vi "子VI-查看某框-不显示界面.vi"(0 "框号":dbl format="%#_13g", 1 "框组":T4(array[cluster]), 2 "临界Z值":i32, 3 "反射图原始路径":path, 4 "临界面积百分比值":dbl, 5 "预先配置的灰度阈值":dbl, 6 "穿透图原始路径":path, 7 "部位信息":string[](array[string])=["", "34.500000", "32.500000", "1121", "34", "54.955926", "分层类", "不合格", ""], 12 "产品规格":cluster{"产品长度（周长）（mm）":dbl, "产品宽度（母线长）（mm）":dbl}) -> (14 "全部检测结果":string[][](table))   [LabVIEW 2018]
uses:
  <vilib>/vision/NI_Vision_Development_Module.lvlib
panel:
  out "弥散类检测结果":string[][](table)
  out "?":string[][](table)
  in  "格式字符串 4":string="%f"
  in  "分隔符（'\\'代码显示） 3":string="\t"
  out "Particle Reports (Pixels)":T1(array[cluster]) {"Orientation" format="%.2f"; "Dimensions"."Height" format="%.2f"; "Dimensions"."Width" format="%.2f"; "Center of Mass"."Y" format="%.2f"; "Center of Mass"."X" format="%.2f"; "Bounding Rect"."Bottom" format="%.2f"; "Bounding Rect"."Right" format="%.2f"; "Bounding Rect"."Top" format="%.2f"; "Bounding Rect"."Left" format="%.2f"; "Number of Holes" format="%.2f"; "Area" format="%.2f"}
  in  "格式字符串 3":string="%f"
  in  "分隔符（'\\'代码显示） 2":string="\t"
  out "弥散缺陷个数":i32
  out "分层缺陷个数":i32
  out "合格？ 弥散类":string="fencengThreshold"
  out "合格？分层类":string="fencengThreshold"
  in  "Tab Control":T2
  out "穿透ROI":T3(plugin-control)
  out "Threshold Image":T3(plugin-control)
  out "?":T3(plugin-control)
  out "?":T3(plugin-control)
  out "Threshold Image":T3(plugin-control)
  out "Threshold Image":T3(plugin-control)
  out "面积 (pixels)":i32
  in  "格式字符串 2":string="%f"
  in  "分隔符（'\\'代码显示）":string="\t"
  # "所选区域信息"
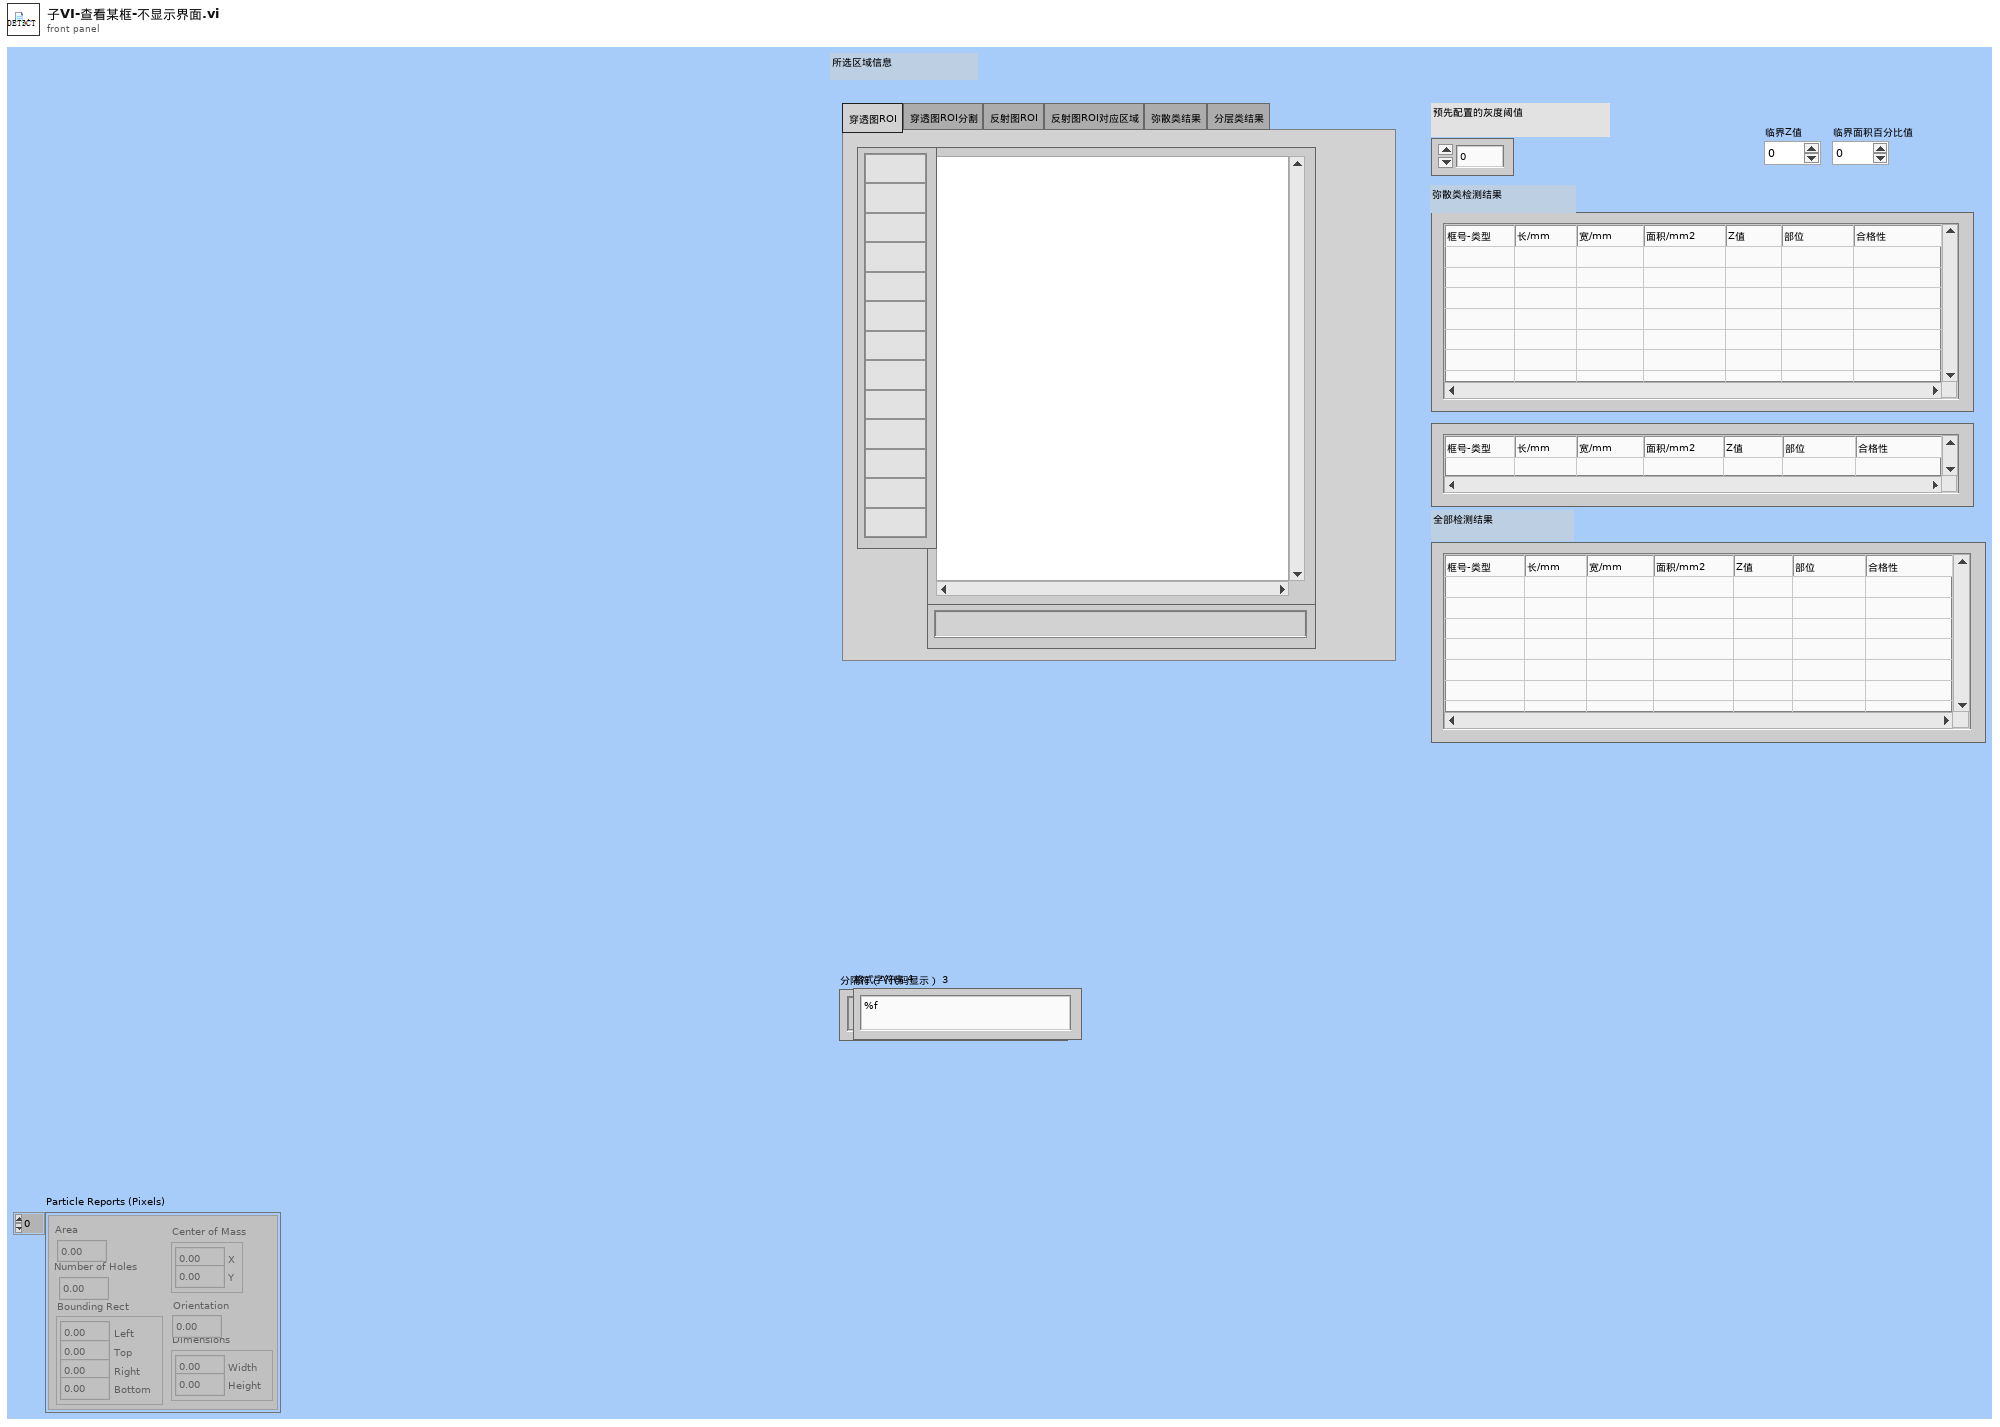
[diagram p1: front panel]
types:
  T1 = cluster{"Area":dbl, "Number of Holes":dbl, "Bounding Rect":cluster{"Left":dbl, "Top":dbl, "Right":dbl, "Bottom":dbl}, "Center of Mass":cluster{"X":dbl, "Y":dbl}, "Orientation":dbl, "Dimensions":cluster{"Width":dbl, "Height":dbl}}[]
  T2 = typedef "控件 1.ctl" = enum32{"穿透图ROI", "穿透图ROI分割", "反射图ROI", "反射图ROI对应区域", "弥散类结果", "分层类结果"}
  T3 = typedef "IMAQ Image.ctl" = refnum<image>
  T4 = cluster{"Global Rectangle":i32[], "Contours":cluster{"Contour Type":u32, "ROI Type":u32, "Points":i32[]}[]}[]
  T5 = typedef "Image Type" = u32
  T6 = cluster{"Global Rectangle":i32[], "Contours":cluster{"Contour Type":u32, "ROI Type":u32, "Points":i32[]}[]}
  T7 = cluster{"histogram":u32[], "Minimal Value":sgl, "Maximal Value":sgl, "Starting Value":sgl, "Interval Width":sgl, "Mean Value":sgl, "Standard  Variation":sgl, "Area (pixels)":i32}
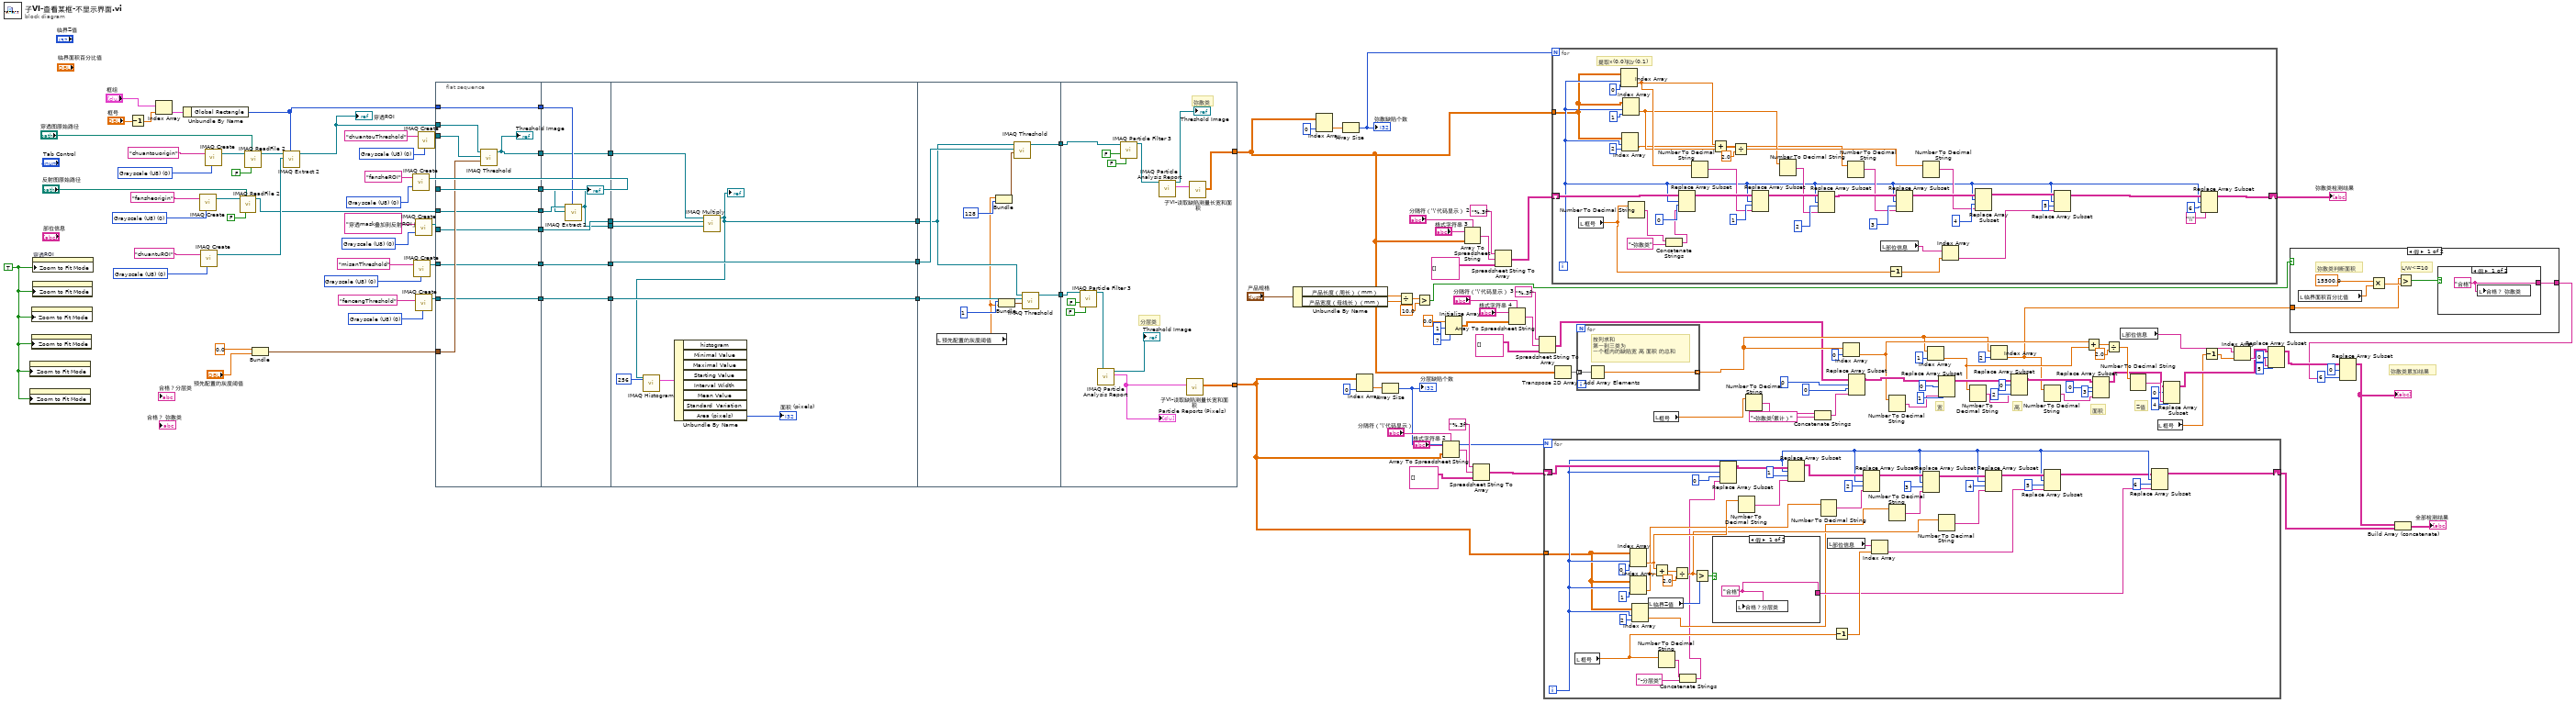
[diagram p0: block diagram]
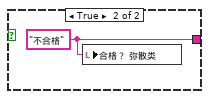
[diagram p2: hidden frame]
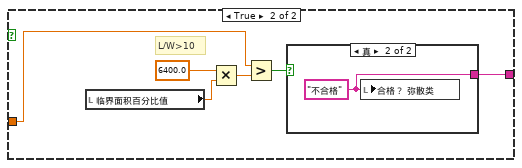
[diagram p3: hidden frame]
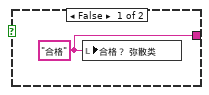
[diagram p4: hidden frame]
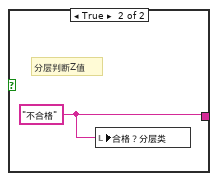
[diagram p5: hidden frame]
diagram:
  w108 = T5 0 items=["Grayscale (U8)", "Grayscale (I16)", "Grayscale (SGL)", "Complex (CSG)", "RGB (U32)", "HSL (U32)", "RGB (U64)", "Grayscale (U16)"] ("Image Type")
  w109 = T5 0 items=["Grayscale (U8)", "Grayscale (I16)", "Grayscale (SGL)", "Complex (CSG)", "RGB (U32)", "HSL (U32)", "RGB (U64)", "Grayscale (U16)"] ("Image Type")
  w110 = T5 0 items=["Grayscale (U8)", "Grayscale (I16)", "Grayscale (SGL)", "Complex (CSG)", "RGB (U32)", "HSL (U32)", "RGB (U64)", "Grayscale (U16)"] ("Image Type")
  w114 = T5 0 items=["Grayscale (U8)", "Grayscale (I16)", "Grayscale (SGL)", "Complex (CSG)", "RGB (U32)", "HSL (U32)", "RGB (U64)", "Grayscale (U16)"] ("Image Type")
  w118 = T5 0 items=["Grayscale (U8)", "Grayscale (I16)", "Grayscale (SGL)", "Complex (CSG)", "RGB (U32)", "HSL (U32)", "RGB (U64)", "Grayscale (U16)"] ("Image Type")
  w129 = T5 0 items=["Grayscale (U8)", "Grayscale (I16)", "Grayscale (SGL)", "Complex (CSG)", "RGB (U32)", "HSL (U32)", "RGB (U64)", "Grayscale (U16)"] ("Image Type")
  w102 = T5 0 items=["Grayscale (U8)", "Grayscale (I16)", "Grayscale (SGL)", "Complex (CSG)", "RGB (U32)", "HSL (U32)", "RGB (U64)", "Grayscale (U16)"] ("Image Type")
  w133 = T5 0 items=["Grayscale (U8)", "Grayscale (I16)", "Grayscale (SGL)", "Complex (CSG)", "RGB (U32)", "HSL (U32)", "RGB (U64)", "Grayscale (U16)"] ("Image Type")
  w141 = TRUE ("Zoom to Fit Mode")
  # "弥散类累加结果"
  # "Z值"
  # "面积"
  # "高"
  # "宽"
  n1 = property class="ImageControl"("Zoom to Fit Mode"=w141) -> ()  [unwired: 2 in, 2 out]
  n2 = property class="ImageControl"("Zoom to Fit Mode"=w141) -> ()  [unwired: 2 in, 2 out]
  n3 = property class="ImageControl"("Zoom to Fit Mode"=w141) -> ()  [unwired: 2 in, 2 out]
  n4 = property class="ImageControl"("Zoom to Fit Mode"=w141) -> ()  [unwired: 2 in, 2 out]
  n5 = property class="ImageControl"("Zoom to Fit Mode"=w141) -> ()  [unwired: 2 in, 2 out]
  n6 = property on="穿透ROI" class="ImageControl"("Zoom to Fit Mode"=w141) -> ()  [unwired: 2 in, 2 out]
  n7 = Decrement(x="框号") -> (x-1=w135:dbl)
  n8 = Index Array(array="框组", index=w135) -> (element=w136:T6)
  n9 = Unbundle By Name(w136) -> ("Global Rectangle"=w101:i32[])
  n10 = call "IMAQ Create"("Image Name"="fansheorigin", "Image Type"=w114) -> ("New Image"=w113:T3)  [unwired: 3 in, 1 out]
  n11 = call "IMAQ Create"("Image Name"="chuantuROI", "Image Type"=w118) -> ("New Image"=w117:T3)  [unwired: 3 in, 1 out]
  n12 = call "IMAQ Create"("Image Name"="chuantouorigin", "Image Type"=w133) -> ("New Image"=w120:T3)  [unwired: 3 in, 1 out]
  n13 = call "IMAQ ReadFile 2"("Use File Path Image Type"=FALSE, "File Path"="反射图原始路径", "Image"=w113) -> ("Image Out"=w97:T3)  [unwired: 4 in, 4 out]
  n14 = call "IMAQ ReadFile 2"("Use File Path Image Type"=FALSE, "File Path"="穿透图原始路径", "Image"=w120) -> ("Image Out"=w121:T3)  [unwired: 4 in, 4 out]
  n15 = Bundle(0.0, "预先配置的灰度阈值"="预先配置的灰度阈值") -> (w76:cluster{dbl, "预先配置的灰度阈值":dbl})  [unwired: 1 in]
  n16 = call "IMAQ Extract 2"("Optional Rectangle"=w101, "Image Dst"=w117, "Image Src"=w121) -> ("Image Dst Out"=w99:T3)  [unwired: 7 in, 1 out]
  "穿透ROI" <- w99
  n17 = call "IMAQ Create"("Image Name"="fansheROI", "Image Type"=w102) -> ("New Image"=w98:T3)  [unwired: 3 in, 1 out]
  n18 = call "IMAQ Create"("Image Name"="misanThreshold", "Image Type"=w108) -> ("New Image"=w84:T3)  [unwired: 3 in, 1 out]
  n19 = call "IMAQ Create"("Image Name"="穿透mask叠加到反射ROI上", "Image Type"=w129) -> ("New Image"=w92:T3)  [unwired: 3 in, 1 out]
  n20 = call "IMAQ Create"("Image Name"="fencengThreshold", "Image Type"=w109) -> ("New Image"=w82:T3)  [unwired: 3 in, 1 out]
  n21 = call "IMAQ Create"("Image Name"="chuantouThreshold", "Image Type"=w110) -> ("New Image"=w100:T3)  [unwired: 3 in, 1 out]
  n22 = flat-sequence {
    tunnel: w101 -> [w151]
    tunnel: w100 -> [w150]
    tunnel: w99 -> [w149]
    tunnel: w76 -> [w148]
    tunnel: w98 -> [w147]
    tunnel: w97 -> [w146]
    tunnel: [w151] -> w96
    tunnel: [w147] -> w95
    tunnel: [w146] -> w94
    tunnel: [w145] -> w93
    tunnel: w92 -> [w145]
    tunnel: [w144] -> w89
    tunnel: w84 -> [w143]
    tunnel: [w143] -> w86
    tunnel: [w142] -> w83
    tunnel: w82 -> [w142]
    tunnel: w96 -> [w159]
    tunnel: w95 -> [w152]
    tunnel: w94 -> [w153]
    tunnel: w93 -> [w158]
    tunnel: [w158] -> w91
    tunnel: [w157] -> w90
    tunnel: w89 -> [w157]
    tunnel: [w156] -> w88
    tunnel: w86 -> [w155]
    tunnel: [w155] -> w85
    tunnel: w83 -> [w154]
    tunnel: [w154] -> w81
    tunnel: w91 -> [w168]
    tunnel: w90 -> [w167]
    tunnel: w88 -> [w166]
    tunnel: [w165] -> w87
    tunnel: w85 -> [w165]
    tunnel: w81 -> [w164]
    tunnel: [w164] -> w80
    tunnel: [w160] -> w79
    tunnel: w87 -> [w178]
    tunnel: w80 -> [w177]
    tunnel: w79 -> [w176]
    tunnel: [w175] -> w78
    tunnel: [w174] -> w77
    tunnel: [w182] -> w50
    tunnel: [w183] -> w70
    tunnel: w78 -> [w187]
    tunnel: w77 -> [w188]
    frame #0 {
      n23 = call "IMAQ Threshold"("Range"=w148, "Image Dst"=w150, "Image Src"=w149) -> ("Image Dst Out"=w144:T3)  [unwired: 3 in, 5 out]
      "Threshold Image" <- w144
    }
    frame #1 {
      n24 = call "IMAQ Extract 2"("Optional Rectangle"=w159, "Image Dst"=w152, "Image Src"=w153) -> ("Image Dst Out"=w156:T3)  [unwired: 7 in, 1 out]
      "?" <- w156
    }
    frame #2 {
      n25 = call "IMAQ Multiply"("Image Src A"=w167, "Image Dst"=w168, "Image Src B"=w166) -> ("Image Dst Out"=w160:T3)  [unwired: 4 in, 1 out]
      "?" <- w160
      n26 = call "IMAQ Histogram"("Number of Classes"=256, "Image"=w160) -> ("Histogram Report"=w162:T7)  [unwired: 8 in, 1 out]
      n27 = Unbundle By Name(w162) -> ("Area (pixels)"=→"面积 (pixels)":i32)  [unwired: 7 out]
    }
    frame #3 {
      n28 = local read "预先配置的灰度阈值"() -> (w169:dbl)
      n29 = Bundle("预先配置的灰度阈值"=w169, 128) -> (w173:cluster{"预先配置的灰度阈值":dbl, i32})  [unwired: 1 in]
      n30 = Bundle(1, "预先配置的灰度阈值"=w169) -> (w172:cluster{i32, "预先配置的灰度阈值":dbl})  [unwired: 1 in]
      n31 = call "IMAQ Threshold"("Range"=w173, "Image Dst"=w178, "Image Src"=w176) -> ("Image Dst Out"=w174:T3)  [unwired: 3 in, 5 out]
      n32 = call "IMAQ Threshold"("Range"=w172, "Image Dst"=w177, "Image Src"=w176) -> ("Image Dst Out"=w175:T3)  [unwired: 3 in, 5 out]
    }
    frame #4 {
      # "分层类"
      # "弥散类"
      n33 = call "IMAQ Particle Filter 3"("Image Src"=w187, "Keep/Remove Particles (F)"=FALSE, "Reject Border? (F)"=FALSE) -> ("Image Dst Out"=w185:T3)  [unwired: 10 in, 2 out]
      n34 = call "IMAQ Particle Analysis Report"("Image"=w185) -> ("Particle Reports (Pixels)"=w186:T1, "Image Out (duplicate)"=→"Threshold Image":T3)  [unwired: 5 in, 4 out]
      "Particle Reports (Pixels)" <- w186
      n35 = call "IMAQ Particle Filter 3"("Image Src"=w188, "Keep/Remove Particles (F)"=FALSE, "Reject Border? (F)"=FALSE) -> ("Image Dst Out"=w181:T3)  [unwired: 10 in, 2 out]
      n36 = call "IMAQ Particle Analysis Report"("Image"=w181) -> ("Particle Reports (Pixels)"=w179:T1, "Image Out (duplicate)"=→"Threshold Image":T3)  [unwired: 5 in, 4 out]
      n37 = call "子VI-读取缺陷测量长宽和面积.vi"("Particle Reports (Pixels)"=w186) -> ("测量结果"=w183:dbl[][])  [unwired: 10 in]
      n38 = call "子VI-读取缺陷测量长宽和面积.vi"("Particle Reports (Pixels)"=w179) -> ("测量结果"=w182:dbl[][])  [unwired: 10 in]
    }
  }
  n39 = Unbundle By Name("产品规格") -> ("产品长度（周长）（mm）"=w124:dbl, "产品宽度（母线长）（mm）"=w123:dbl)
  n40 = Index Array(array=w50, index (col)=0 ("禁用的索引 (列)")) -> (element=w105:dbl[])  [unwired: 1 in]
  n41 = Array Size(array=w105) -> (size(s)=w62:i32)
  "弥散缺陷个数" <- w62
  n42 = Index Array(array=w70, index (col)=0 ("禁用的索引 (列)")) -> (element=w107:dbl[])  [unwired: 1 in]
  n43 = Array Size(array=w107) -> (size(s)=w68:i32)
  "分层缺陷个数" <- w68
  n44 = Divide(x=w124, y=w123) -> (x/y=w127:dbl)
  n45 = Greater?(x=w127, y=10.0) -> (0:w7:bool)
  n46 = Array To Spreadsheet String(delimiter (Tab)="分隔符（'\\'代码显示）", array=w70, 3:"格式字符串 2") -> (spreadsheet string=w73:string)
  n47 = Initialize Array(0.0 ("元素"), 1 ("维数大小"), 7 ("维数大小")) -> (w52:dbl[][])
  n48 = Array To Spreadsheet String(delimiter (Tab)="分隔符（'\\'代码显示） 2", array=w50, 3:"格式字符串 3") -> (spreadsheet string=w65:string)
  n49 = Spreadsheet String To Array(format string="%.3f", spreadsheet string=w73, array type (2D Dbl)=string[][] [] ("Array")) -> (array=w69:string[][])  [unwired: 1 in]
  n50 = Spreadsheet String To Array(format string="%.3f", spreadsheet string=w65, array type (2D Dbl)=string[][] [] ("Array")) -> (array=w61:string[][])  [unwired: 1 in]
  n51 = Array To Spreadsheet String(delimiter (Tab)="分隔符（'\\'代码显示） 3", array=w52, 3:"格式字符串 4") -> (spreadsheet string=w55:string)
  n52 = Spreadsheet String To Array(format string="%.3f", spreadsheet string=w55, array type (2D Dbl)=string[][] [] ("Array")) -> (array=w23:string[][])  [unwired: 1 in]
  n53 = for {
    N: w68 -> [_]
    tunnel: w70 -> [w198]
    shift-right: [w207] -> w3
    shift-left: w69 -> [w216]
    i -> [w199]
    n54 = local read "框号"() -> (w223:dbl)
    n55 = Index Array(array=w198, index (row)=w199, index (col)=0 ("禁用的索引 (列)")) -> (element=w206:dbl)
    n56 = Index Array(array=w198, index (row)=w199, index (col)=1 ("禁用的索引 (列)")) -> (element=w205:dbl)
    n57 = Index Array(array=w198, index (row)=w199, index (col)=2 ("索引 (列)")) -> (element=w197:dbl)
    n58 = local read "临界Z值"() -> (w230:i32)
    n59 = Add(x=w206, y=w205) -> (x+y=w231:dbl)
    n60 = Number To Decimal String(number=w223) -> (decimal integer string=w195:string)  [unwired: 1 in]
    n61 = Divide(x=w231, y=2.0) -> (x/y=w203:dbl)
    n62 = Concatenate Strings(w195, "-分层类" ("新元素/子数组")) -> (w194:string)
    n63 = Greater?(x=w203, y=w230) -> (0:w232:bool)
    n64 = case shown="假" w232 {
      tunnel: [w233 w234] -> w201
      frame False {
        w233 = "合格" ("合格？")
        n65 = local write "合格？分层类"(w233) -> ()
      }
      frame True {
        w234 = "不合格" ("合格？")
        # "分层判断Z值"
        n66 = local write "合格？分层类"(w234) -> ()
      }
    }
    n67 = Replace Array Subset(array=w216, new element=w194, index (row)=w199, index (col)=0 ("索引 (列)")) -> (w215:string[][])
    n68 = Number To Decimal String(number=w206) -> (decimal integer string=w214:string)  [unwired: 1 in]
    n69 = Replace Array Subset(array=w215, new element=w214, index (row)=w199, index (col)=1 ("索引 (列)")) -> (w212:string[][])
    n70 = Number To Decimal String(number=w205) -> (decimal integer string=w213:string)  [unwired: 1 in]
    n71 = local read "部位信息"() -> (w226:string[])
    n72 = Decrement(x=w223) -> (x-1=w225:dbl)
    n73 = Replace Array Subset(array=w212, new element=w213, index (row)=w199, index (col)=2 ("索引 (列)")) -> (w211:string[][])
    n74 = Index Array(array=w226, index=w225) -> (element=w202:string)
    n75 = Number To Decimal String(number=w197) -> (decimal integer string=w210:string)  [unwired: 1 in]
    n76 = Replace Array Subset(array=w211, new element=w210, index (row)=w199, index (col)=3 ("索引 (列)")) -> (w209:string[][])
    n77 = Number To Decimal String(number=w203) -> (decimal integer string=w204:string)  [unwired: 1 in]
    n78 = Replace Array Subset(array=w209, new element=w204, index (row)=w199, index (col)=4 ("索引 (列)")) -> (w208:string[][])
    n79 = Replace Array Subset(array=w208, new element=w202, index (row)=w199, index (col)=5 ("索引 (列)")) -> (w193:string[][])
    n80 = Replace Array Subset(array=w193, new element=w201, index (row)=w199, index (col)=6 ("索引 (列)")) -> (w207:string[][])
  }
  n81 = for {
    N: w62 -> [_]
    shift-right: [w257] -> w1
    shift-left: w61 -> [w263]
    tunnel: w50 -> [w239]
    i -> [w240]
    # "提取x(0,0)和y(0,1)"
    n82 = local read "框号"() -> (w247:dbl)
    n83 = Index Array(array=w239, index (row)=w240, index (col)=0 ("禁用的索引 (列)")) -> (element=w245:dbl)
    n84 = Index Array(array=w239, index (row)=w240, index (col)=2 ("索引 (列)")) -> (element=w238:dbl)
    n85 = Index Array(array=w239, index (row)=w240, index (col)=1 ("禁用的索引 (列)")) -> (element=w244:dbl)
    n86 = Number To Decimal String(number=w247) -> (decimal integer string=w236:string)  [unwired: 1 in]
    n87 = Concatenate Strings(w236, "-弥散类" ("新元素/子数组")) -> (w235:string)
    n88 = Replace Array Subset(array=w263, new element=w235, index (row)=w240, index (col)=0 ("索引 (列)")) -> (w262:string[][])
    n89 = Number To Decimal String(number=w245) -> (decimal integer string=w256:string)  [unwired: 1 in]
    n90 = Add(x=w245, y=w244) -> (x+y=w253:dbl)
    n91 = Divide(x=w253, y=2.0) -> (x/y=w251:dbl)
    n92 = Replace Array Subset(array=w262, new element=w256, index (row)=w240, index (col)=1 ("索引 (列)")) -> (w261:string[][])
    n93 = Number To Decimal String(number=w244) -> (decimal integer string=w255:string)  [unwired: 1 in]
    n94 = Replace Array Subset(array=w261, new element=w255, index (row)=w240, index (col)=2 ("索引 (列)")) -> (w260:string[][])
    n95 = Number To Decimal String(number=w238) -> (decimal integer string=w254:string)  [unwired: 1 in]
    n96 = local read "部位信息"() -> (w249:string[])
    n97 = Decrement(x=w247) -> (x-1=w248:dbl)
    n98 = Replace Array Subset(array=w260, new element=w254, index (row)=w240, index (col)=3 ("索引 (列)")) -> (w259:string[][])
    n99 = Number To Decimal String(number=w251) -> (decimal integer string=w250:string)  [unwired: 1 in]
    n100 = Index Array(array=w249, index=w248) -> (element=w246:string)
    n101 = Replace Array Subset(array=w259, new element=w250, index (row)=w240, index (col)=4 ("索引 (列)")) -> (w258:string[][])
    n102 = Replace Array Subset(array=w258, new element=w246, index (row)=w240, index (col)=5 ("索引 (列)")) -> (w243:string[][])
    n103 = Replace Array Subset(array=w243, new element="\\" ("新元素/子数组"), index (row)=w240, index (col)=6 ("索引 (列)")) -> (w257:string[][])
  }
  "弥散类检测结果" <- w1
  n104 = Transpose 2D Array(2D array=w50) -> (transposed array=w51:dbl[][])
  n105 = for {
    tunnel: w51 -> [w274] mode=indexing
    tunnel: [w273] -> w24 mode=indexing
    # "按列求和 \n第一到三类为\n一个框内的缺陷宽 高 面积 的总和"
    n106 = Add Array Elements(numeric array=w274) -> (sum=w273:dbl)
  }
  n107 = local read "框号"() -> (w25:dbl)
  n108 = Number To Decimal String(number=w25) -> (decimal integer string=w28:string)  [unwired: 1 in]
  n109 = Concatenate Strings(w28, "-弥散类(累计）" ("新元素/子数组")) -> (w26:string)
  n110 = Index Array(array=w24, index=0 ("索引")) -> (element=w30:dbl)
  n111 = Replace Array Subset(array=w23, new element=w26, index (row)=0 ("禁用的索引 (行)"), index (col)=0 ("索引 (列)")) -> (w44:string[][])
  n112 = Number To Decimal String(number=w30) -> (decimal integer string=w43:string)  [unwired: 1 in]
  n113 = Index Array(array=w24, index=1 ("索引")) -> (element=w29:dbl)
  n114 = Replace Array Subset(array=w44, new element=w43, index (row)=0 ("索引 (行)"), index (col)=1 ("索引 (列)")) -> (w41:string[][])
  n115 = Number To Decimal String(number=w29) -> (decimal integer string=w34:string)  [unwired: 1 in]
  n116 = Index Array(array=w24, index=2 ("索引")) -> (element=w6:dbl)
  n117 = Replace Array Subset(array=w41, new element=w34, index (row)=0 ("索引 (行)"), index (col)=2 ("禁用的索引 (列)")) -> (w36:string[][])
  n118 = Number To Decimal String(number=w6) -> (decimal integer string=w33:string)  [unwired: 1 in]
  n119 = Add(x=w30, y=w29) -> (x+y=w32:dbl)
  n120 = Replace Array Subset(array=w36, new element=w33, index (row)=0 ("索引 (行)"), index (col)=3 ("索引 (列)")) -> (w11:string[][])
  n121 = Divide(x=w32, y=2.0) -> (x/y=w12:dbl)
  n122 = local read "部位信息"() -> (w10:string[])
  n123 = Number To Decimal String(number=w12) -> (decimal integer string=w22:string)  [unwired: 1 in]
  n124 = local read "框号"() -> (w8:dbl)
  n125 = Replace Array Subset(array=w11, new element=w22, index (row)=0 ("索引 (行)"), index (col)=4 ("索引 (列)")) -> (w9:string[][])
  n126 = Decrement(x=w8) -> (x-1=w19:dbl)
  n127 = Index Array(array=w10, index=w19) -> (element=w18:string)
  n128 = Replace Array Subset(array=w9, new element=w18, index (row)=0 ("索引 (行)"), index (col)=5 ("索引 (列)")) -> (w13:string[][])
  n129 = case shown="假" w7 {
    tunnel: [w279 w285] -> w5
    tunnel: w6 -> [w275 w283]
    frame False {
      # "弥散类判断面积"
      # "L/W<=10"
      n130 = local read "临界面积百分比值"() -> (w277:dbl)
      n131 = Multiply(x=15500.0, y=w277) -> (x*y=w276:dbl)
      n132 = Greater?(x=w275, y=w276) -> (0:w280:bool)
      n133 = case shown="假" w280 {
        tunnel: [w281 w282] -> w279
        frame False {
          w281 = "合格" ("合格？")
          n134 = local write "合格？ 弥散类"(w281) -> ()
        }
        frame True {
          w282 = "不合格" ("合格？")
          n135 = local write "合格？ 弥散类"(w282) -> ()
        }
      }
    }
    frame True {
      # "L/W>10"
      n136 = local read "临界面积百分比值"() -> (w286:dbl)
      n137 = Multiply(x=6400.0, y=w286) -> (x*y=w284:dbl)
      n138 = Greater?(x=w283, y=w284) -> (0:w288:bool)
      n139 = case shown="真" w288 {
        tunnel: [w289 w290] -> w285
        frame False {
          w289 = "合格" ("合格？")
          n140 = local write "合格？ 弥散类"(w289) -> ()
        }
        frame True {
          w290 = "不合格" ("合格？")
          n141 = local write "合格？ 弥散类"(w290) -> ()
        }
      }
    }
  }
  n142 = Replace Array Subset(array=w13, new element=w5, index (row)=0 ("索引 (行)"), index (col)=6 ("索引 (列)")) -> (w2:string[][])
  "?" <- w2
  n143 = Build Array (concatenate)(w2, w3) -> (→"全部检测结果":string[][])
